vi "GEA2 HEWH ERDs.vi"(7 "Enable Diagnostic Data":T1, 8 "Error In":errorcluster, 9 "Disable ERD (Main)":bool, 10 "LV Program":T2, 11 "Disable Electronic Mixing Valve (EMV) List":bool) -> (0 "Error Out":errorcluster, 1 "Read ERD List":T4[](array[typedef]) {"ERD Number" format="%.0x"}, 2 "GEA Inputs":T3 {"Destination" format="%.0x"; "Source" format="%.0x"}, 3 "ERD Headers":string[](array[string]))   [LabVIEW 2016]
uses:
  type defs/ERD Read Data In.ctl
  type defs/Data Type.ctl
  type defs/Source_Destination.ctl
  Save File/File Setup (Public)/Type Definition/Save File DOE LabView Program.ctl
  Washer HCC/Washer HCC NEWFI/Type Definitions/HCC Washer Types.ctl
  library/GEA2_Toolkit.lvlib
  Save File/File Setup.lvlib
panel:
  in  "Tab Control":enum32{"HEWH", "Washer"}(tab)
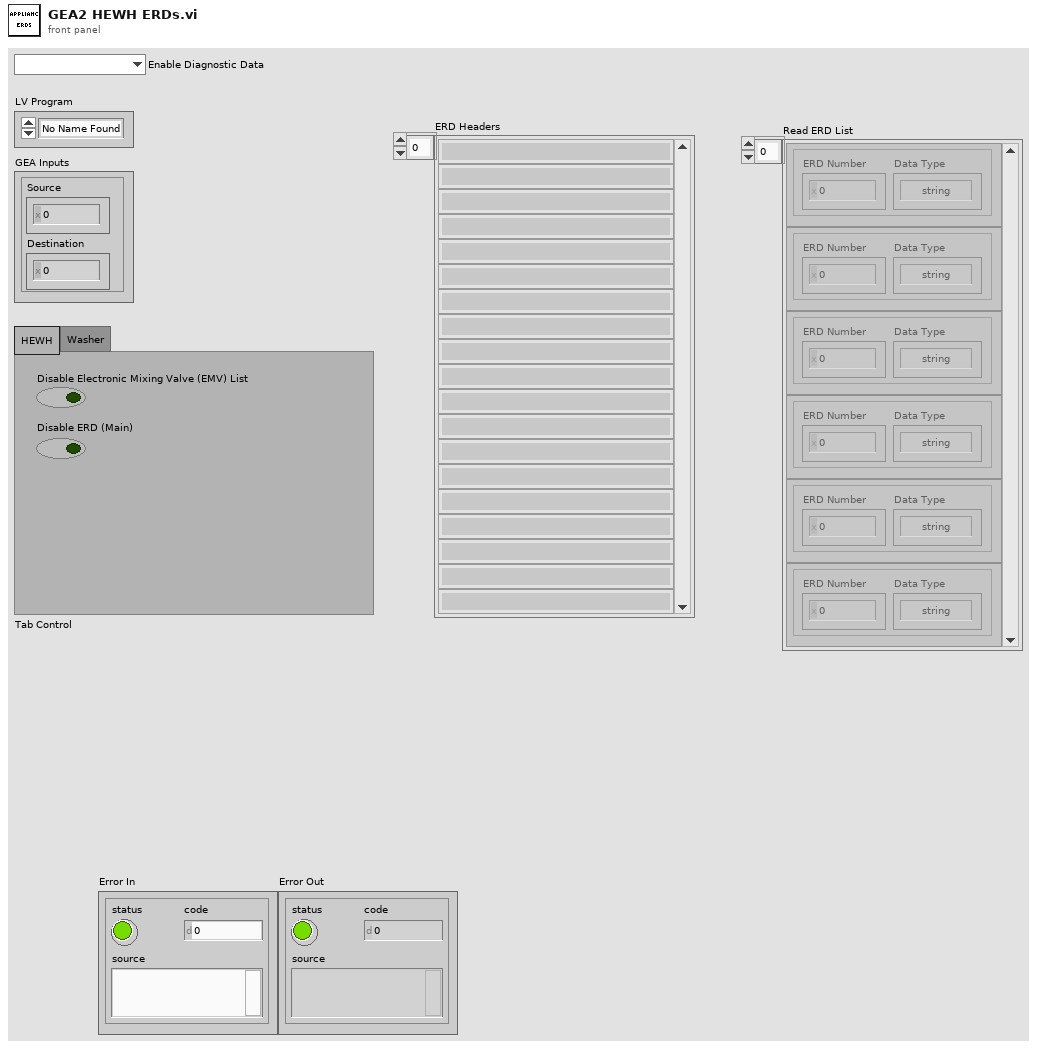
[diagram p1: front panel]
types:
  T1 = typedef "HCC Washer Types.ctl" = enum16{"", "Viper Washer", "Hawk Washer", "2015 Washer", "2017 Washer"}
  T2 = typedef "File Setup.lvlib/Save File DOE LabView Program.ctl" = enum16{"No Name Found", "DOE Stand", "Dishwasher Kitchen", "Portable Stand", "HEWH", "Dryer", "Dryer WILT", "HCC", "PRAT", "HEWH RLT", "Refrigeration"}
  T3 = typedef "GEA2_Toolkit.lvlib/Source_Destination.ctl" = cluster{"Source":u8, "Destination":u8}
  T4 = typedef "GEA2_Toolkit.lvlib/ERD Read Data In.ctl" = cluster{"ERD Number":u16, "Data Type":T5}
  T5 = typedef "GEA2_Toolkit.lvlib/Data Type.ctl" = enum16{"string", "boolean", "uint8_t", "uint16_t", "uint32_t", "uint64_t"}
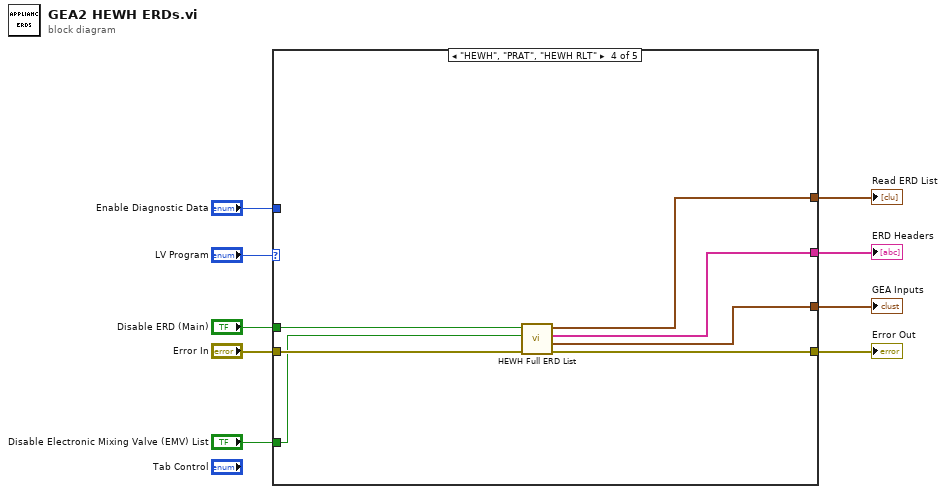
[diagram p0: block diagram]
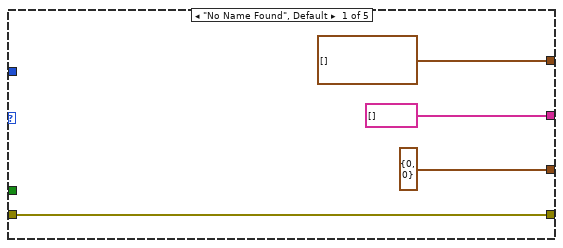
[diagram p2: hidden frame]
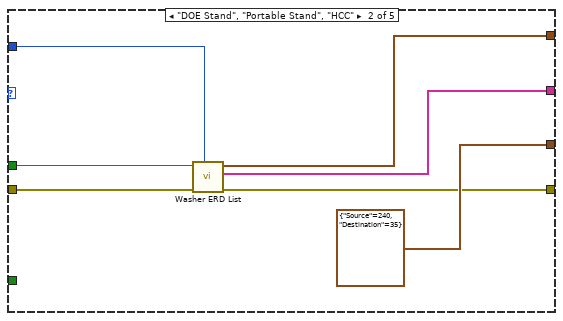
[diagram p3: hidden frame]
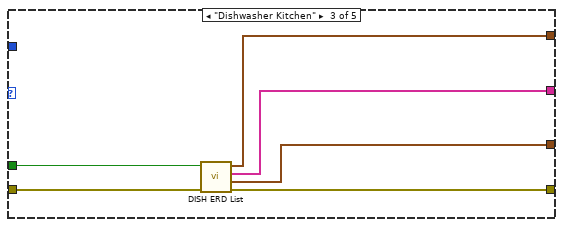
[diagram p4: hidden frame]
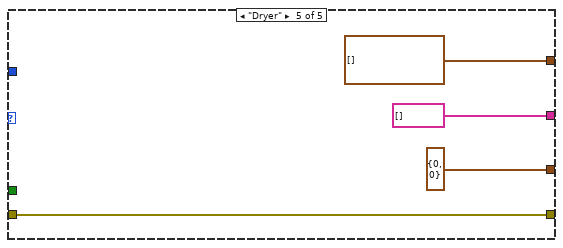
[diagram p5: hidden frame]
diagram:
  n1 = case shown="\"HEWH\", \"PRAT\", \"HEWH RLT\"" "LV Program" {
    tunnel: [string[] [] w20 w25 w31 string[] []] -> w1
    tunnel: [T4[] [] ("Read ERD List") w19 w24 w30 T4[] [] ("Read ERD List")] -> w5
    tunnel: [T3 {"Source"=0, "Destination"=0} ("GEA Inputs") T3 {"Source"=240, "Destination"=35} ("GEA Inputs") w26 w33 T3 {"Source"=0, "Destination"=0} ("GEA Inputs")] -> w9
    tunnel: [w13 w15 w21 w32 w36] -> w8
    tunnel: "Error In" -> [w13 w16 w22 w28 w36]
    tunnel: "Disable ERD (Main)" -> [_ w18 w23 w29 _]
    tunnel: "Enable Diagnostic Data" -> [_ w14 _ _ _]
    tunnel: "Disable Electronic Mixing Valve (EMV) List" -> [_ _ _ w27 _]
    frame "No Name Found", Default {
    }
    frame "DOE Stand", "Portable Stand", "HCC" {
      n2 = call "Washer ERD List.vi"("Enable Diagnostic Data"=w14, "Error In"=w16, "Disable ERD (Main)"=w18) -> ("Error Out"=w15:errorcluster, "Header Array"=w20:string[], "Read ERD List"=w19:T4[])  [unwired: 6 in]
    }
    frame "Dishwasher Kitchen" {
      n3 = call "DISH ERD List.vi"("Error In"=w22, "Disable ERD (Main)"=w23) -> ("Error Out"=w21:errorcluster, "GEA Inputs"=w26:T3, "Array"=w25:string[], "Read ERD List"=w24:T4[])  [unwired: 6 in]
    }
    frame "HEWH", "PRAT", "HEWH RLT" {
      n4 = call "HEWH Full ERD List.vi"("error in (no error)"=w28, "Disable Electronic Mixing Valve (EMV) List"=w27, "Disable ERD (Main)"=w29) -> ("error out"=w32:errorcluster, "GEA Inputs"=w33:T3, "ERD Headers"=w31:string[], "Read ERD List"=w30:T4[])  [unwired: 5 in]
    }
    frame "Dryer" {
    }
  }
  "ERD Headers" <- w1
  "Read ERD List" <- w5
  "GEA Inputs" <- w9
  "Error Out" <- w8
